vi "RW From File.vi"(8 "error in":errorcluster, 10 "Mode":string="rb", 11 "File":string="c:\\temp\\hello.bmp") -> (0 "error out":errorcluster, 3 "RWops Pointer":u32 format="%.0x")   [LabVIEW 2015, in "LibSDL2.lvlib"]
uses:
  LibSDL2.lvlib
  DLL/SDL2.dll
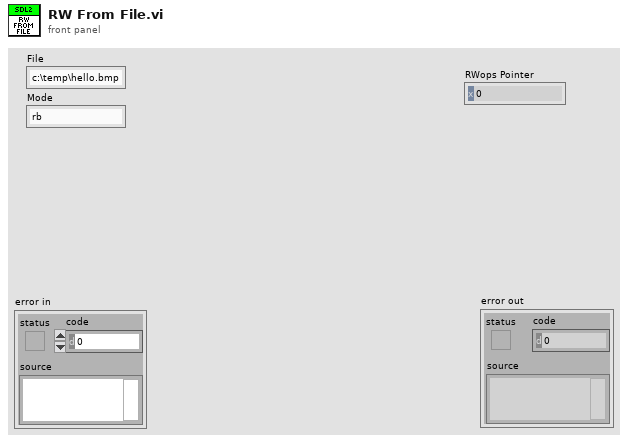
[diagram p1: front panel]
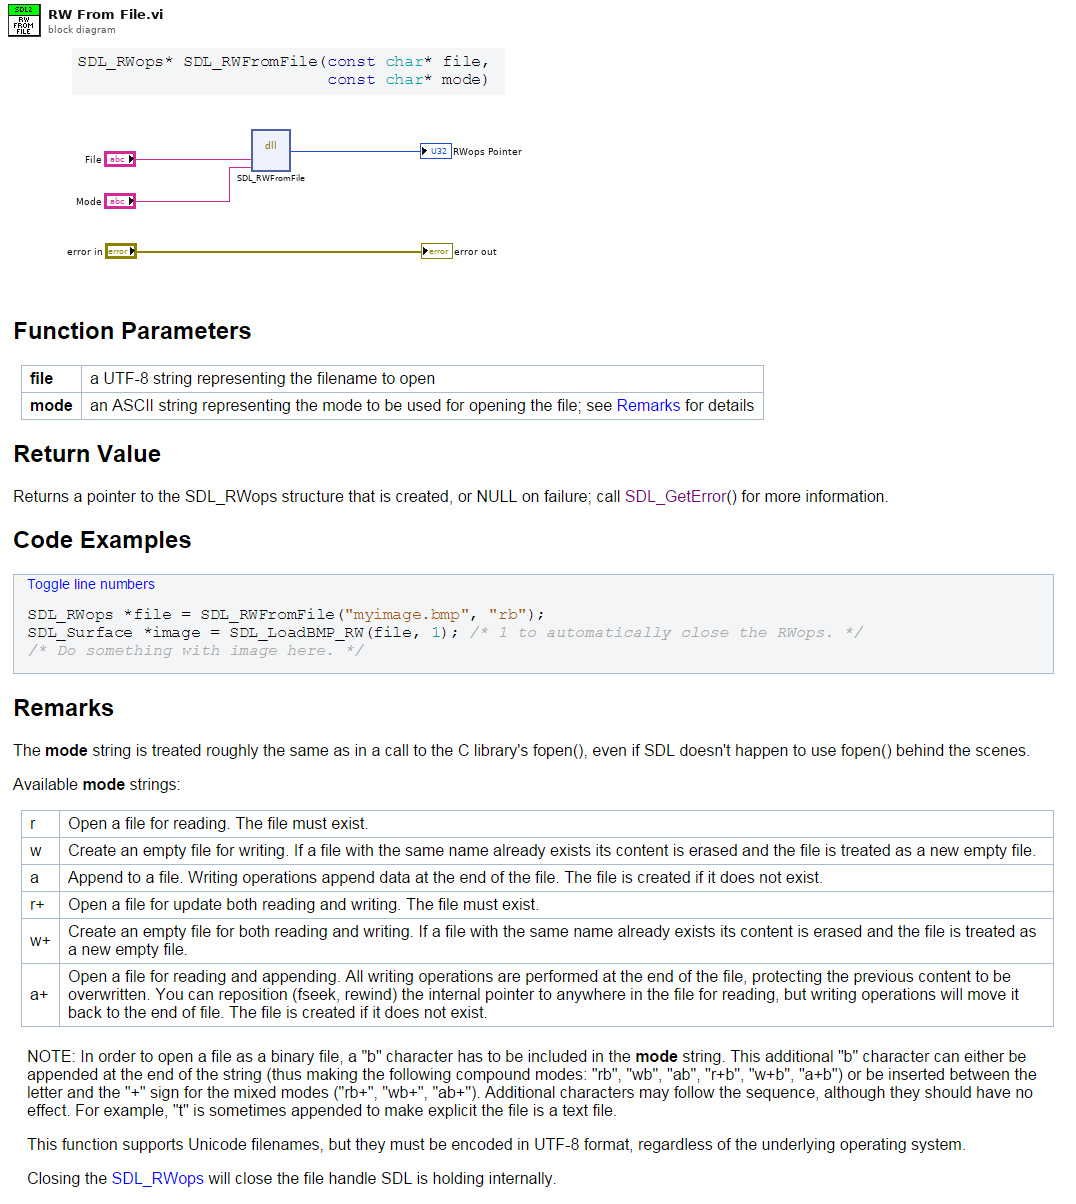
[diagram p0: block diagram]
diagram:
  n1 = dll-call lib="C:/dev/PGS/LabSDL2/Source/Libraries/LibSDL2 Wrapper/DLL/SDL2.dll" fn="SDL_RWFromFile"("file"="File", "mode"="Mode") -> ("return type"=→"RWops Pointer":u32)  [unwired: 5 in, 2 out]
  "error out" <- "error in"
